vi "PXI Multipliers to AO Gains (1D).vi"(0 "Multipliers in":dbl[](array[numeric]), 11 "error in (no error)":errorcluster) -> (4 "Multipliers out":dbl[](array[numeric]), 6 "Gains":dbl[](array[numeric]), 15 "error out":errorcluster)   [LabVIEW 2020]
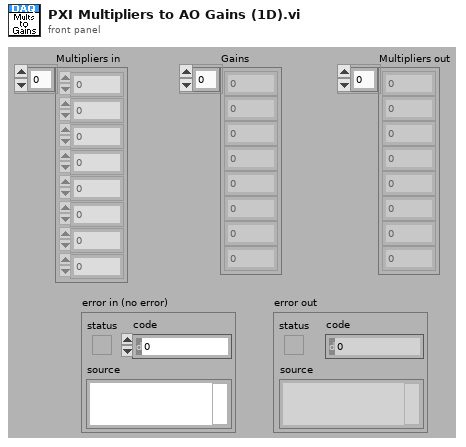
[diagram p1: front panel]
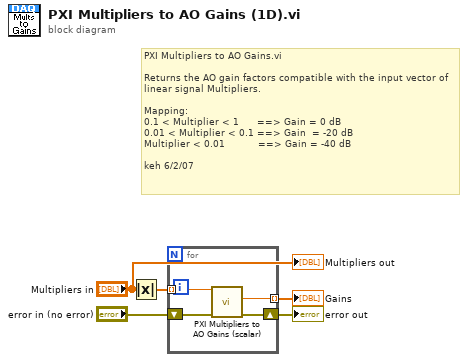
[diagram p0: block diagram]
diagram:
  # "PXI Multipliers to AO Gains.vi\n\nReturns the AO gain factors compatible with the input vector of linear signal Multipliers.\n\nMapping:\n0.1 < Multiplier < 1      ==> Gain = 0 dB\n0.01 < Multiplier < 0.1 ==> Gain  = -20 dB\nMultiplier < 0.01           ==> Gain = -40 dB\n\nkeh 6/2/07"
  n1 = Absolute Value(x="Multipliers in") -> (abs(x)=w5:dbl[])
  n2 = for {
    tunnel: [w8] -> w4 mode=indexing
    tunnel: w5 -> [w9] mode=indexing
    shift-right: [w6] -> w2
    shift-left: "error in (no error)" -> [w7]
    n3 = call "PXI Multipliers to AO Gains (scalar).vi"("Multiplier In"=w9, "error in (no error)"=w7) -> ("Gain"=w8:dbl, "error out"=w6:errorcluster)  [unwired: 11 in, 1 out]
  }
  "Gains" <- w4
  "error out" <- w2
  "Multipliers out" <- "Multipliers in"
